vi "Display Confirmation to User.vi"(7 "Confirmation Type":T2, 8 "error in (no error)":errorcluster, 11 "Config":T1) -> (0 "error out":errorcluster, 1 "New Config?":bool, 2 "OK?":bool, 3 "Config out":T1)   [LabVIEW 2023, in "VI Properties Editor.lvlib"]
doc: "Displays a confirmation dialog to the user, taking into account <B>Confirmation Type</B> and <B>Config</B>."
uses:
  VI Properties Editor.lvlib
  CTLs/Confirmation Type.ctl
  CTLs/Config.ctl
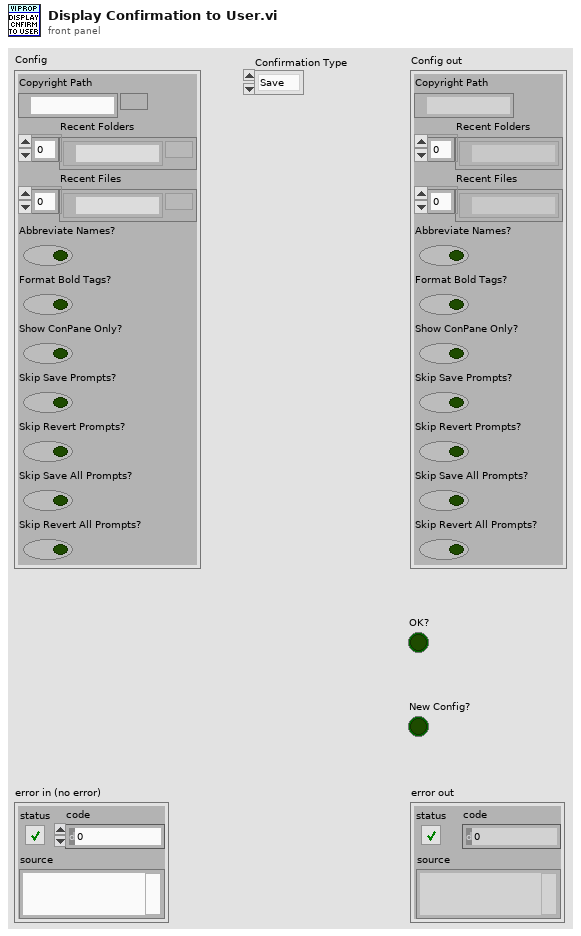
[diagram p1: front panel]
types:
  T1 = typedef "VI Properties Editor.lvlib/Config.ctl" = cluster{"Copyright Path":path, "Recent Folders":path[], "Recent Files":path[], "Abbreviate Names?":bool, "Format Bold Tags?":bool, "Show ConPane Only?":bool, "Skip Save Prompts?":bool, "Skip Revert Prompts?":bool, "Skip Save All Prompts?":bool, "Skip Revert All Prompts?":bool}
  T2 = typedef "VI Properties Editor.lvlib/Confirmation Type.ctl" = enum16{"Save", "Save All", "Revert", "Revert All"}
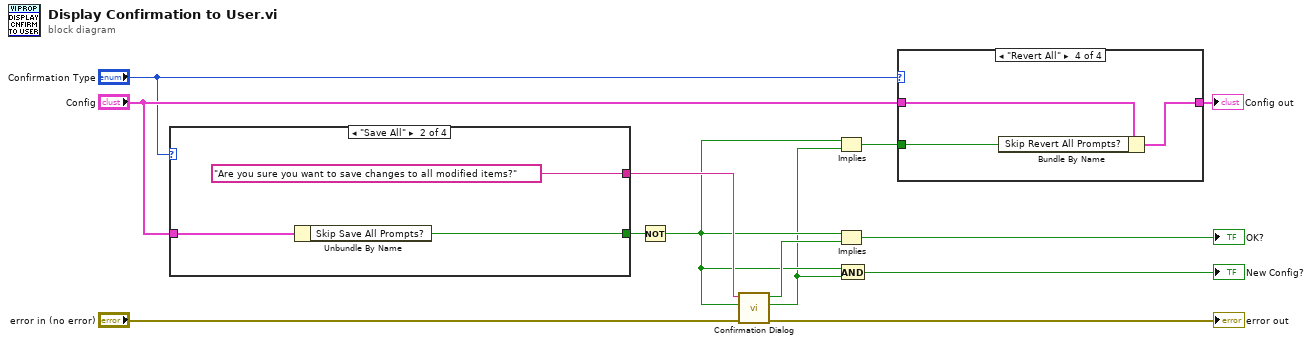
[diagram p0: block diagram]
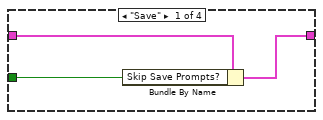
[diagram p2: hidden frame]
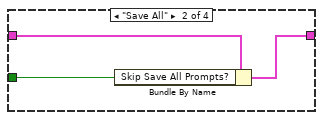
[diagram p3: hidden frame]
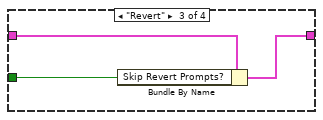
[diagram p4: hidden frame]
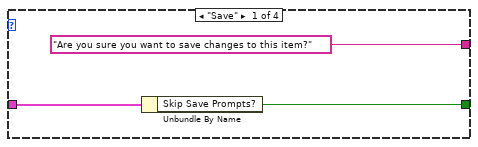
[diagram p5: hidden frame]
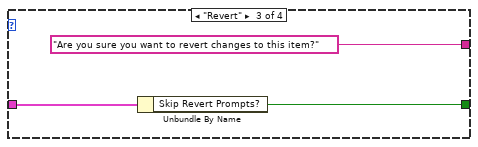
[diagram p6: hidden frame]
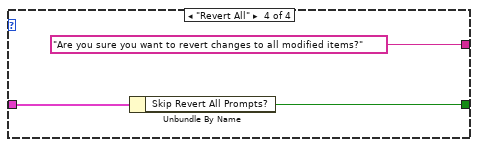
[diagram p7: hidden frame]
diagram:
  n1 = case shown="\"Save All\"" "Confirmation Type" {
    tunnel: ["Are you sure you want to save changes to this item?" "Are you sure you want to save changes to all modified items?" "Are you sure you want to revert changes to this item?" "Are you sure you want to revert changes to all modified items?"] -> w11
    tunnel: "Config" -> [w15 w18 w21 w24]
    tunnel: [w14 w17 w20 w23] -> w10
    frame "Save" {
      n2 = Unbundle By Name(w15) -> ("Skip Save Prompts?"=w14:bool)
    }
    frame "Save All" {
      n3 = Unbundle By Name(w18) -> ("Skip Save All Prompts?"=w17:bool)
    }
    frame "Revert" {
      n4 = Unbundle By Name(w21) -> ("Skip Revert Prompts?"=w20:bool)
    }
    frame "Revert All" {
      n5 = Unbundle By Name(w24) -> ("Skip Revert All Prompts?"=w23:bool)
    }
  }
  n6 = Not(x=w10) -> (.not. x?=w3:bool)
  n7 = call "Confirmation Dialog.vi"("error in (no error)"="error in (no error)", "Enable"=w3, "Message"=w11) -> ("error out"=→"error out":errorcluster, "Skip Prompts?"=w2:bool, "OK?"=w4:bool)  [unwired: 6 in]
  n8 = Implies(1:w2, 2:w3) -> (0:w6:bool)
  n9 = Implies(1:w4, 2:w3) -> (0:→"OK?":bool)
  n10 = And(x=w3, y=w2) -> (x .and. y?=→"New Config?":bool)
  n11 = case shown="\"Revert All\"" "Confirmation Type" {
    tunnel: "Config" -> [w28 w31 w34 w37]
    tunnel: [w27 w30 w33 w36] -> w5
    tunnel: w6 -> [w26 w29 w32 w35]
    frame "Save" {
      n12 = Bundle By Name(cluster=w28, "Skip Save Prompts?"=w26) -> (w27:T1)
    }
    frame "Save All" {
      n13 = Bundle By Name(cluster=w31, "Skip Save All Prompts?"=w29) -> (w30:T1)
    }
    frame "Revert" {
      n14 = Bundle By Name(cluster=w34, "Skip Revert Prompts?"=w32) -> (w33:T1)
    }
    frame "Revert All" {
      n15 = Bundle By Name(cluster=w37, "Skip Revert All Prompts?"=w35) -> (w36:T1)
    }
  }
  "Config out" <- w5
